vi "_TEST Steps.vi"(4 "error in (no error)":errorcluster) -> (0 "error out":errorcluster)   [LabVIEW 2011]
uses:
  Step Record.ctl
  Sequences/Sequence Record.ctl
panel:
  out "Sequence Steps":T1[](array[typedef])
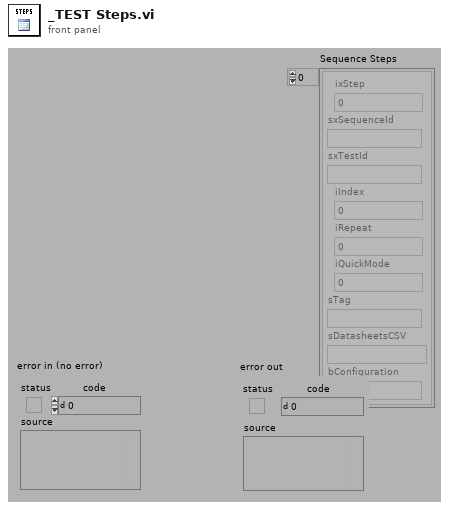
[diagram p1: front panel]
types:
  T1 = typedef "Step Record.ctl" = cluster{"ixStep":i32, "sxSequenceId":string, "sxTestId":string, "iIndex":i32, "iRepeat":i32, "iQuickMode":i32, "sTag":string, "sDatasheetsCSV":string, "bConfiguration":string}
  T2 = typedef "Sequence Record.ctl" = cluster{"ixSequence":i32, "sxSequenceId":string, "sDescription":string, "sCreator":string, "tCreationDate":timestamp, "sModifier":string, "tModifiedDate":timestamp, "fApproved":bool, "fSpartanSetsSN":bool, "fOverwriteData":bool, "fStopOnFail":bool, "fDisableQuickMode":bool, "fPartialExecution":bool, "fAutoNextItem":bool, "fDoNotPrintOnFail":bool}
  T3 = typedef "Connection Refnum.ctl" = cluster{"Environment Handle":i32, "Connection Handle":i32}
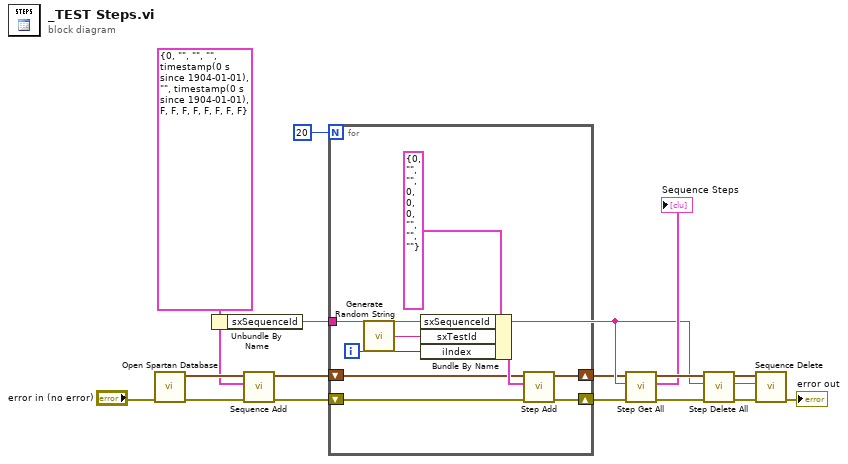
[diagram p0: block diagram]
diagram:
  w14 = T2 {"ixSequence"=0, "sxSequenceId"="", "sDescription"="", "sCreator"="", "tCreationDate"=timestamp(0 s since 1904-01-01), "sModifier"="", "tModifiedDate"=timestamp(0 s since 1904-01-01), "fApproved"=FALSE, "fSpartanSetsSN"=FALSE, "fOverwriteData"=FALSE, "fStopOnFail"=FALSE, "fDisableQuickMode"=FALSE, "fPartialExecution"=FALSE, "fAutoNextItem"=FALSE, "fDoNotPrintOnFail"=FALSE} ("Sequence Record")
  n1 = call "Open Spartan Database.vi"("error in (no error)"="error in (no error)") -> ("error out"=w15:errorcluster, "Connection Refnum"=w16:T3)  [unwired: 1 in, 8 out]
  n2 = Unbundle By Name(w14) -> ("sxSequenceId"=w7:string)
  n3 = call "Sequence Add.vi"("error in (no error)"=w15, "Sequence Record"=w14, "Connection Refnum"=w16) -> ("error out"=w4:errorcluster, "Connection Refnum"=w2:T3)  [unwired: 7 out]
  n4 = for {
    N: 20 -> [_]
    tunnel: w7 -> [w24]
    shift-right: [w20] -> w3
    shift-left: w4 -> [w21]
    shift-right: [w17] -> w1
    shift-left: w2 -> [w18]
    i -> [w23]
    n5 = call "Generate Random String.vi"() -> ("Output String"=w22:string)  [unwired: 1 in, 4 out]
    n6 = Bundle By Name(cluster=T1 {"ixStep"=0, "sxSequenceId"="", "sxTestId"="", "iIndex"=0, "iRepeat"=0, "iQuickMode"=0, "sTag"="", "sDatasheetsCSV"="", "bConfiguration"=""} ("Sequence Step Record"), "sxSequenceId"=w24, "sxTestId"=w22, "iIndex"=w23) -> (w19:T1)
    n7 = call "Step Add.vi"("error in (no error)"=w21, "Step Record"=w19, "Connection Refnum"=w18) -> ("error out"=w20:errorcluster, "Connection Refnum"=w17:T3)  [unwired: 6 in, 1 out]
  }
  n8 = call "Step Get All.vi"("error in (no error)"=w3, "sxSequenceId"=w7, "Connection Refnum"=w1) -> ("error out"=w11:errorcluster, "Sequence Steps"=→"Sequence Steps":T1[], "Connection Refnum"=w12:T3)  [unwired: 1 in, 5 out]
  n9 = call "Step Delete All.vi"("error in (no error)"=w11, "sxSequenceId (\"\")"=w7, "Connection Refnum"=w12) -> ("error out"=w8:errorcluster, "Connection Refnum"=w9:T3)  [unwired: 7 out]
  n10 = call "Sequence Delete.vi"("error in (no error)"=w8, "Sequence ID"=w7, "Connection Refnum"=w9) -> ("error out"=→"error out":errorcluster)  [unwired: 8 out]
